vi "Set Brower UI Refs.vi"(8 "error in (no error)":errorcluster, 10 "Brower UI Refs":T1, 11 "BrowerController in":refnum<class "BrowerController.lvclass">) -> (0 "error out":errorcluster, 3 "BrowerController out":refnum<class "BrowerController.lvclass">)   [LabVIEW 2015, in "BrowerController.lvclass"]
uses:
  BrowerController.lvclass
  Type Definition/Brower UI Refs.ctl
  BrowerController.lvclass/BrowerController.ctl
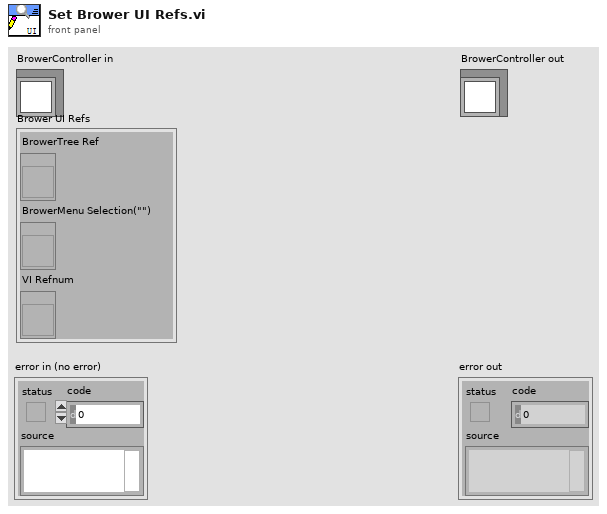
[diagram p1: front panel]
types:
  T1 = typedef "BrowerController.lvclass/Brower UI Refs.ctl" = cluster{"BrowerTree Ref":refnum<vi>, "BrowerMenu Selection(\"\")":refnum<vi>, "VI Refnum":refnum<vi>}
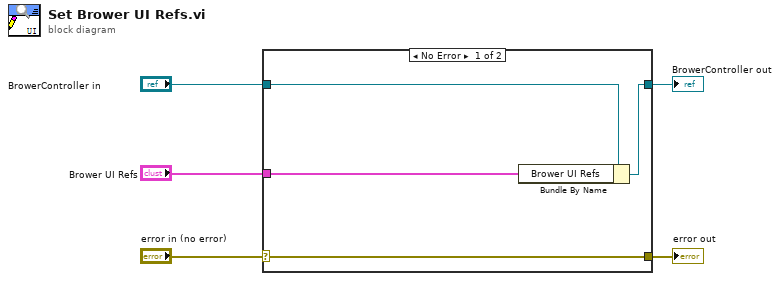
[diagram p0: block diagram]
diagram:
  n1 = case shown="No Error" "error in (no error)" {
    selector: "error in (no error)" -> [w9 w10]
    tunnel: [w9 w10] -> w4
    tunnel: [w7 w11] -> w2
    tunnel: "BrowerController in" -> [w8 w11]
    tunnel: "Brower UI Refs" -> [w6 _]
    frame No Error {
      n2 = Bundle By Name(cluster=w8, "Brower UI Refs"=w6) -> (w7:refnum<class "BrowerController.lvclass">)
    }
    frame Error {
    }
  }
  "error out" <- w4
  "BrowerController out" <- w2
